vi "9.7.vi"() -> ()   [LabVIEW 2017]
panel:
  out "output":dbl
  in  "input":dbl
  in  "Enum":enum16{"f to c", "c to f"}(ring)
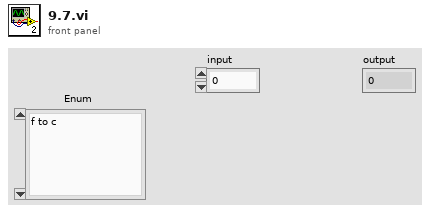
[diagram p1: front panel]
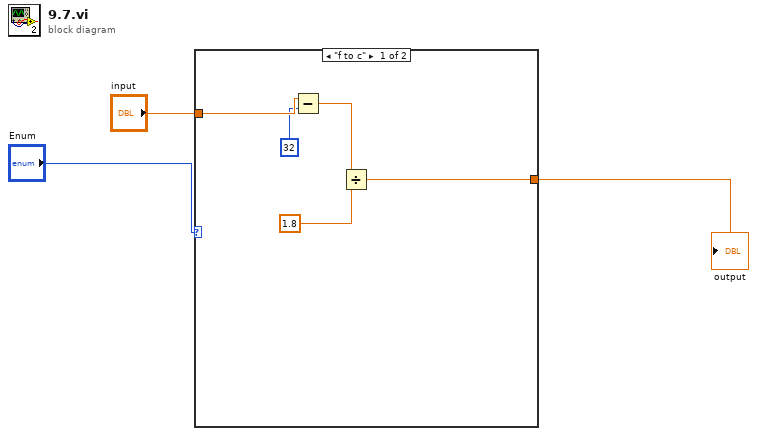
[diagram p0: block diagram]
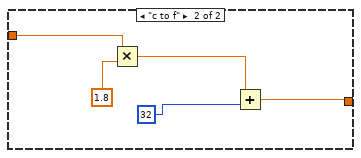
[diagram p2: hidden frame]
diagram:
  n1 = case shown="\"f to c\"" "Enum" {
    tunnel: "input" -> [w8 w12]
    tunnel: [w4 w10] -> w1
    frame "f to c" {
      n2 = Subtract(x=w8, y=32) -> (x-y=w6:dbl)
      n3 = Divide(x=w6, y=1.8) -> (x/y=w4:dbl)
    }
    frame "c to f" {
      n4 = Multiply(x=w12, y=1.8) -> (x*y=w11:dbl)
      n5 = Add(x=w11, y=32) -> (x+y=w10:dbl)
    }
  }
  "output" <- w1
